vi "Iterative Initial Position.vi"(8 "error in (no error)":errorcluster, 9 "Number of\nLBCBs In":T1, 10 "Act Cmds In":dbl[][](array[numeric])) -> (0 "error out":errorcluster, 2 "Cmd Out":T2[](array[typedef]))   [LabVIEW 2013]
uses:
  Act & Cart Commands.ctl
  Data Access Objects/Application/Number Of LBCBs.ctl
panel:
  out "Reconstituted Act Cmds":dbl[][](array[numeric])
  out "Act Error":dbl[][](array[numeric])
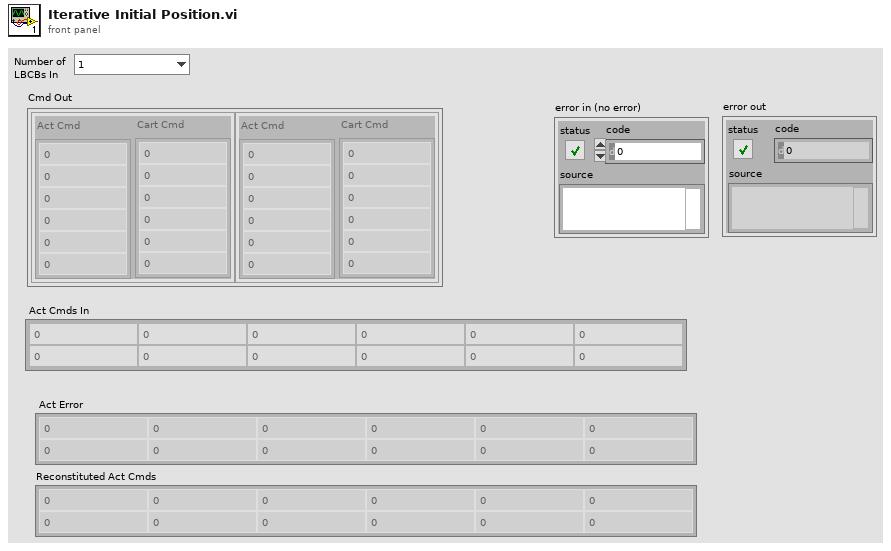
[diagram p1: front panel]
types:
  T1 = typedef "Number Of LBCBs.ctl" = enum16{"1", "2"}
  T2 = typedef "Act & Cart Commands.ctl" = cluster{"Act Cmd":dbl[], "Cart Cmd":dbl[]}
  T3 = enum16{"Cartesian2ActuatorDisplacements", "Actuator2CartesianDisplacements", "Actuators2CartesianForces"}
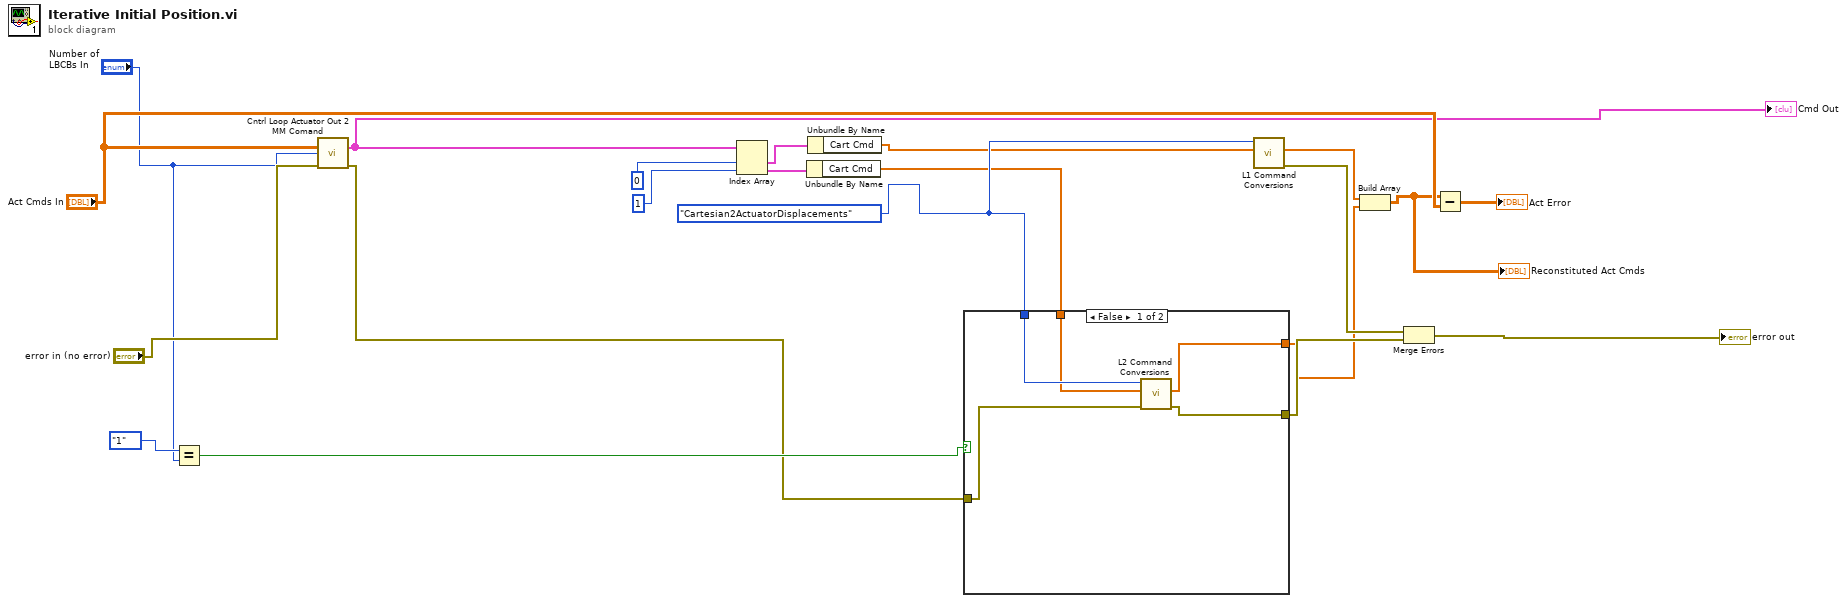
[diagram p0: block diagram]
diagram:
  w17 = T3."Cartesian2ActuatorDisplacements" ("ConversionOps")
  n1 = Equal?(x=Number_Of_LBCBs."1", y="Number of\nLBCBs In") -> (x = y?=w18:bool)
  n2 = call "Cntrl Loop Actuator Out 2 MM Comand.vi"("Act Cmds In"="Act Cmds In", "Number of\nLBCBs In"="Number of\nLBCBs In", "error in (no error)"="error in (no error)") -> ("Cmd Out"=w2:T2[], "error out"=w4:errorcluster)  [unwired: 11 in]
  "Cmd Out" <- w2
  n3 = Index Array(array=w2, index #1=0 ("index"), index #2=1 ("index")) -> (element #1=w14:T2, element #2=w10:T2)
  n4 = Unbundle By Name(w10) -> ("Cart Cmd"=w9:dbl[])
  n5 = Unbundle By Name(w14) -> ("Cart Cmd"=w13:dbl[])
  n6 = case shown="False" w18 {
    tunnel: w9 -> [w25 w28]
    tunnel: [w22 w28] -> w7
    tunnel: w4 -> [w24 w27]
    tunnel: [w23 w27] -> w12
    tunnel: w17 -> [w26 _]
    frame False {
      n7 = call "L2 Command Conversions.vi"("error in (no error)"=w24, "Inputs"=w25, "ConversionOps"=w26) -> ("error out"=w23:errorcluster, "Outputs"=w22:dbl[])  [unwired: 7 in]
    }
    frame True {
    }
  }
  n8 = call "L1 Command Conversions.vi"("Inputs"=w13, "ConversionOps"=w17) -> ("error out"=w11:errorcluster, "Outputs"=w8:dbl[])  [unwired: 8 in]
  n9 = Build Array(w8, w7) -> (w1:dbl[][])
  "Reconstituted Act Cmds" <- w1
  n10 = Merge Errors(w11, w12) -> (→"error out":errorcluster)
  n11 = Subtract(x=w1, y="Act Cmds In") -> (x-y=→"Act Error":dbl[][])
